vi "parse_scanner_data.vi"(6 "batch_active?":bool, 7 "DOCK_gear_serial":refnum<vi>, 10 "SCANNER_data":string, 11 "all_config_info":T1 {"main_ini_file"."SCANNER Flow control" items=["None"=0, "XON/XOFF"=1, "RTS/CTS"=2, "DTR/DSR"=4]; "main_ini_file"."SCANNER Stop bits" items=["1.0"=10, "1.5"=15, "2.0"=20]}) -> ()   [LabVIEW 2019]
uses:
  ini/typedef/DOCK_all_config_info.ctl
  ini/typedef/DOCK_main_ini_file.ctl
  queues/typedef/DOCK_queue_refnums.ctl
  queues/typedef/DOCK_MAIN_queue_element.ctl
  MAIN/DOCK_MAIN_sequence_state.ctl
  queues/typedef/DOCK_SCANNER_queue_element.ctl
  DOCK_SCANNER_sequence_state.ctl
  queues/typedef/DOCK_PRINTER_queue_element.ctl
  PRINTER/DOCK_PRINTER_sequence_state.ctl
  FGV/login/FGV_DOCK_login.ctl
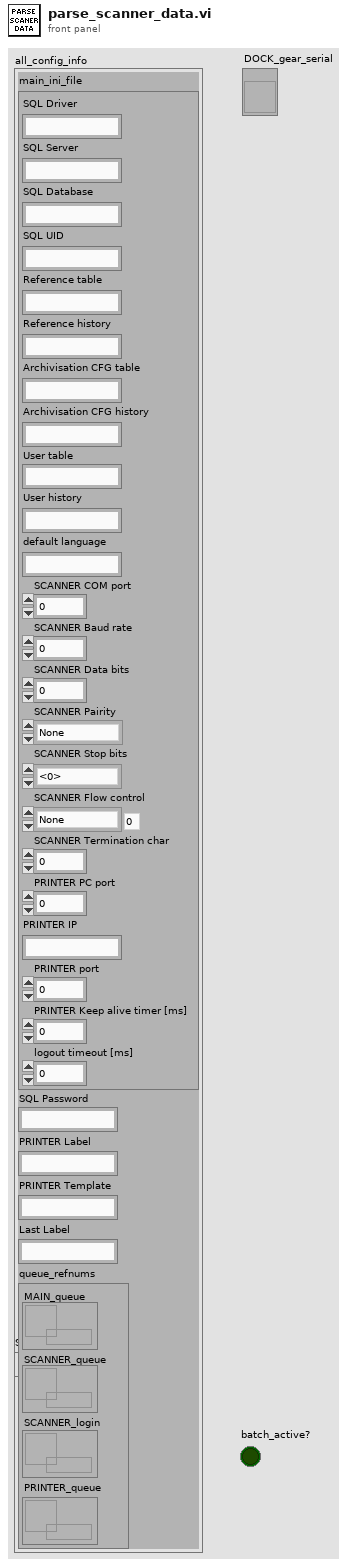
[diagram p1: front panel]
types:
  T1 = typedef "DOCK_all_config_info.ctl" = cluster{"main_ini_file":T2, "SQL Password":string, "PRINTER Label":string, "PRINTER Template":string, "Last Label":string, "queue_refnums":T3}
  T2 = typedef "DOCK_main_ini_file.ctl" = cluster{"SQL Driver":string, "SQL Server":string, "SQL Database":string, "SQL UID":string, "Reference table":string, "Reference history":string, "Archivisation CFG table":string, "Archivisation CFG history":string, "User table":string, "User history":string, "default language":string, "SCANNER COM port":u16, "SCANNER Baud rate":u32, "SCANNER Data bits":u16, "SCANNER Pairity":enum16{"None", "Odd", "Even", "Mark", "Space"}, "SCANNER Stop bits":u16, "SCANNER Flow control":u16, "SCANNER Termination char":u8, "PRINTER PC port":u16, "PRINTER IP":string, "PRINTER port":u16, "PRINTER Keep alive timer [ms]":i32, "logout timeout [ms]":i32}
  T3 = typedef "DOCK_queue_refnums.ctl" = cluster{"MAIN_queue":refnum<queue>, "SCANNER_queue":refnum<queue>, "SCANNER_login":refnum<queue>, "PRINTER_queue":refnum<queue>}
  T4 = typedef "FGV_DOCK_login.ctl" = enum16{"initialize", "start_login_read", "end_login_read", "login", "logout", "get_login_info"}
  T5 = typedef "DOCK_MAIN_queue_element.ctl" = cluster{"state":T6, "variable":variant}
  T6 = typedef "DOCK_MAIN_sequence_state.ctl" = enum16{"initialize", "get_next_state", "USER_login", "USER_logout", "read_reference_list", "read_batch_size_list", "change_reference", "start_batch", "reload_batch", "finish_batch?", "finish_batch", "preread_gear_data_check", "read_gear_data", "refresh_gear_data", "save_gear_to_batch", "clear_gear_data", "print_label", "report_get", "error", "stop"}
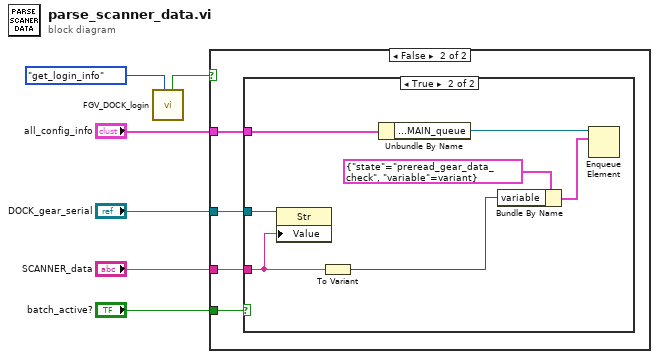
[diagram p0: block diagram]
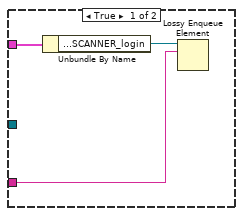
[diagram p2: hidden frame]
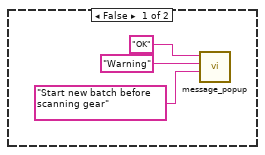
[diagram p3: hidden frame]
diagram:
  n1 = call "FGV_DOCK_login.vi"("options"=FGV_DOCK_login."get_login_info") -> ("Login read active?"=w5:bool)  [unwired: 6 in, 4 out]
  n2 = case shown="False" w5 {
    tunnel: "all_config_info" -> [w9 w13]
    tunnel: "SCANNER_data" -> [w7 w12]
    tunnel: "DOCK_gear_serial" -> [_ w11]
    tunnel: "batch_active?" -> [_ w10]
    frame True {
      n3 = Unbundle By Name(w9) -> ("queue_refnums.SCANNER_login"=w8:refnum<queue>)
      n4 = Lossy Enqueue Element(queue=w8, element=w7) -> ()  [unwired: 1 in, 4 out]
    }
    frame False {
      n5 = case shown="True" w10 {
        tunnel: w13 -> [_ w23]
        tunnel: w12 -> [_ w18]
        tunnel: w11 -> [_ w17]
        frame False {
          n6 = call "message_popup.vi"("Message"="Start new batch before scanning gear", "Title"="Warning", "Button Label"="OK") -> ()  [unwired: 8 in, 1 out]
        }
        frame True {
          n7 = property class="Str"(reference=w17, "Value"=w18) -> ()  [unwired: 1 in, 2 out]
          n8 = To Variant(anything=w18) -> (Variant=w20:variant)
          n9 = Unbundle By Name(w23) -> ("queue_refnums.MAIN_queue"=w22:refnum<queue>)
          n10 = Bundle By Name(cluster=T5 {"state"=enum."preread_gear_data_check", "variable"=variant} ("element"), "variable"=w20) -> (w21:T5)
          n11 = Enqueue Element(queue=w22, element=w21) -> ()  [unwired: 2 in, 3 out]
        }
      }
    }
  }
